vi "Launch Nested.vi"(7 "ID":string, 8 "error in (no error)":errorcluster, 10 "Nested Actor":refnum<class "Actor.lvclass">, 11 "TEC Controller in":refnum<class "TEC Controller.lvclass">) -> (0 "error out":errorcluster, 3 "TEC Controller out":refnum<class "TEC Controller.lvclass">)   [LabVIEW 2014, in "Humidifier Test Lib.lvlib" / "TEC Controller.lvclass"]
uses:
  TEC Controller.lvclass
  <vilib>/ActorFramework/Actor/Actor.lvclass
  TEC Controller.lvclass/TEC Controller.ctl
  <vilib>/ActorFramework/Message Enqueuer/Message Enqueuer.lvclass
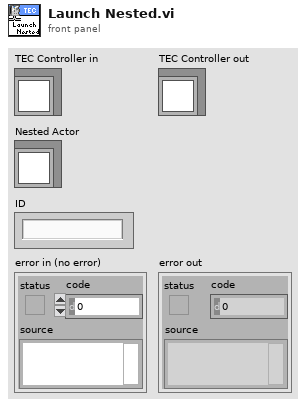
[diagram p1: front panel]
types:
  T1 = cluster{"Enqueuer":refnum<class "Message Enqueuer.lvclass">, "Active":bool}
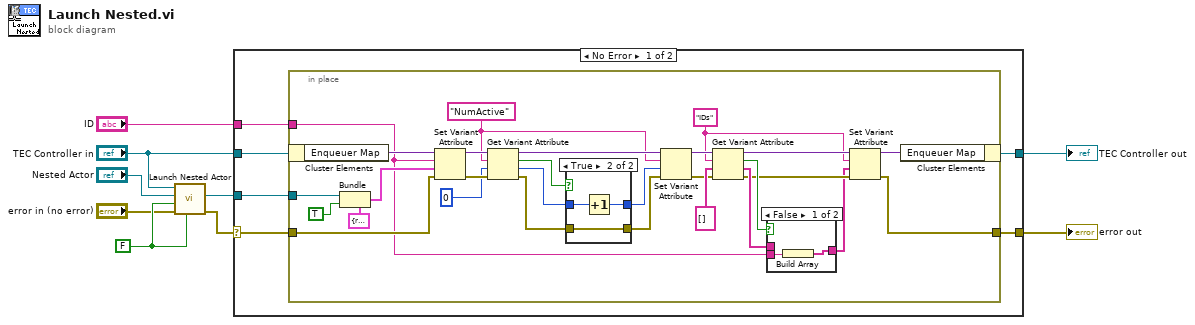
[diagram p0: block diagram]
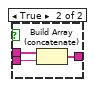
[diagram p2: hidden frame]
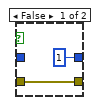
[diagram p3: hidden frame]
diagram:
  w7 = FALSE ("Open Actor Core front panel? (F)")
  n1 = call <vilib>:"Launch Nested Actor.vi"("Open Actor Core front panel? (F)"=w7, "error in (no error)"="error in (no error)", "Auto-stop? (T)"=w7, "Nested Actor"="Nested Actor", "Caller Actor in"="TEC Controller in") -> ("error out"=w8:errorcluster, "Nested Actor's Enqueuer"=w9:refnum<class "Message Enqueuer.lvclass">)  [unwired: 4 in, 1 out]
  n2 = case shown="No Error" w8 {
    selector: w8 -> [w12 w54]
    tunnel: "TEC Controller in" -> [w15 w55]
    tunnel: [w14 w55] -> w1
    tunnel: w9 -> [w13 _]
    tunnel: [w11 w54] -> w2
    tunnel: "ID" -> [w10 _]
    frame No Error {
      n3 = in-place {
        in-place-border: w13 -> [w42]
        in-place-border: w12 -> [w39]
        in-place-border: [w18] -> w11
        in-place-border: w10 -> [w17]
        w19 = "IDs" ("name")
        w30 = "NumActive" ("name")
        n4 = in-place-cluster #1(w15) -> ("Enqueuer Map"=w43:variant)
        n5 = Bundle(cluster=T1 {"Enqueuer"=refnum, "Active"=FALSE} ("eMap"), "Enqueuer"=w42, "Active"=TRUE) -> (w41:T1)
        n6 = Set Variant Attribute(Variant=w43, name=w17, value=w41, error in=w39) -> (Variant out=w37:variant, error out=w38:errorcluster)  [unwired: 1 out]
        n7 = Get Variant Attribute(Variant=w37, name=w30, default value (empty Variant)=i16 0 ("unsigned 8bit integer"), error in=w38) -> (duplicate Variant=w34:variant, found=w33:bool, value=w36:i16, error out=w32:errorcluster)
        n8 = case shown="True" w33 {
          tunnel: w36 -> [_ w51]
          tunnel: [i16 1 w53] -> w35
          tunnel: w32 -> [w49 w52]
          tunnel: [w49 w52] -> w31
          frame False {
          }
          frame True {
            n9 = Increment(x=w51) -> (x+1=w53:i16)
          }
        }
        n10 = Set Variant Attribute(Variant=w34, name=w30, value=w35, error in=w31) -> (Variant out=w28:variant, error out=w26:errorcluster)  [unwired: 1 out]
        n11 = Get Variant Attribute(Variant=w28, name=w19, default value (empty Variant)=string[] [], error in=w26) -> (duplicate Variant=w23:variant, found=w25:bool, value=w24:string[], error out=w21:errorcluster)
        n12 = case shown="False" w25 {
          tunnel: w24 -> [_ w48]
          tunnel: w17 -> [w45 w47]
          tunnel: [w44 w46] -> w20
          frame False {
            n13 = Build Array(w45) -> (w44:string[])
          }
          frame True {
            n14 = Build Array (concatenate)(w48, w47) -> (w46:string[])
          }
        }
        n15 = Set Variant Attribute(Variant=w23, name=w19, value=w20, error in=w21) -> (Variant out=w22:variant, error out=w18:errorcluster)  [unwired: 1 out]
        n16 = in-place-cluster #1("Enqueuer Map"=w22) -> (w14:refnum<class "TEC Controller.lvclass">)
      }
    }
    frame Error {
      # "If the launch fails"
    }
  }
  "error out" <- w2
  "TEC Controller out" <- w1
